vi "Sync Project.vi"() -> ()   [LabVIEW 2011, in "LVH-Build-Tools.lvlib"]
doc: "This VI duplicates the install directories folder hierarchy in the source directory (if neccissary) and creates hard links in the source directory for each new file in the install directory. This VI should be run each time after LabVIEW development, before checking in code."
uses:
  <vilib>/LabVIEW Hacker/Build Tools/LVH-Build-Tools.lvlib
  vi.lib/LabVIEW Hacker/Build Tools/Private/Type Defs/Sync Source State.ctl
panel:
  out "Error Out":errorcluster
  out "Window":enum32{"Init", "Configure", "Sync", "Summary"}(tab)
  in  "Config Help Button":bool
  in  "Settings Button":bool
  in  "Project":u16(ring) items=["LVH-Adept", "LVH-Build-Tools", "LVH-LINX", "LVH-Revert", "LVH-Toolbox"]
  in  "LabVIEW Version":u16(ring) items=["NI LabVIEW 2011 SP1"]
  in  "Config Next Button":bool
  in  "Config Cancel":bool
  out "Progress":picture
  out "Mass Compile Log":string
  out "Added Files":string[](array[string])
  in  "Summary Finish Button":bool
  out "Deleted Files":string[](array[string])
  out "Archive Link":string
  # "Sync Project\nInitializing..."
  # "Sync Project\n\nPlease choose a project to sync and the version of LabVIEW to sync from."
  # "Sync Project\n\nSyncing, please wait..."
  # "Sync Project\n\nSync complete.  Press Finish to exit."
  # "Backup Archive:"
  # "Mass Compile Log"
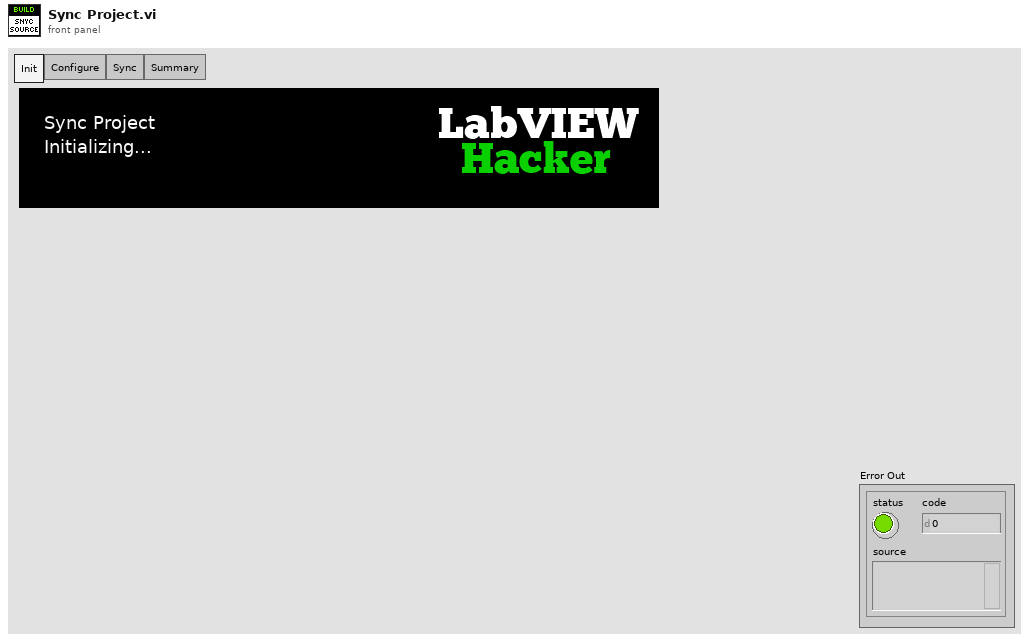
[diagram p1: front panel]
types:
  T1 = typedef "LVH-Build-Tools.lvlib/Sync Source State.ctl" = enum16{"Init", "Configure", "Sync", "Summary"}
  T2 = typedef "LVH-Build-Tools.lvlib/Sync Source Configuration.ctl" = cluster{"Installed Projects":T3[], "Project Source Root Dir":path, "All Config Files":path[], "Selected Project Config":path, "All LabVIEW Dirs":path[], "Selected LabVIEW Dir":path, "Backup Dir":path}
  T3 = typedef "LVH-Build-Tools.lvlib/Installed Project.ctl" = cluster{"Project Name":string, "LV Versions":T4[], "Project Config Path":path}
  T4 = typedef "LVH-Build-Tools.lvlib/_Installed LabVIEW Version.ctl" = cluster{"Version":string, "Path":path}
  T5 = typedef "LVH-Build-Tools.lvlib/_Animation Config.ctl" = cluster{"Image Data":T6[], "Animation Picture Indicator":refnum<vi>, "FPS":u32, "Position":cluster{"X":i16, "Y":i16}}
  T6 = typedef "imagedata.ctl" = cluster{"image type":i32, "image depth":i32, "image":u8[], "mask":u8[], "colors":u32[], "Rectangle":cluster{"left":i16, "top":i16, "right":i16, "bottom":i16}}
  T7 = typedef "LVH-Build-Tools.lvlib/Configuration.ctl" = cluster{"Source Root":path, "Install Root":string, "Components":string[], "Ignore":string[], "Config Files":path[], "LV Directories":path[], "Install Paths":T8}
  T8 = typedef "LVH-Build-Tools.lvlib/Install Configuration.ctl" = cluster{"LabVIEW Directory":path, "Project Source Config":path}
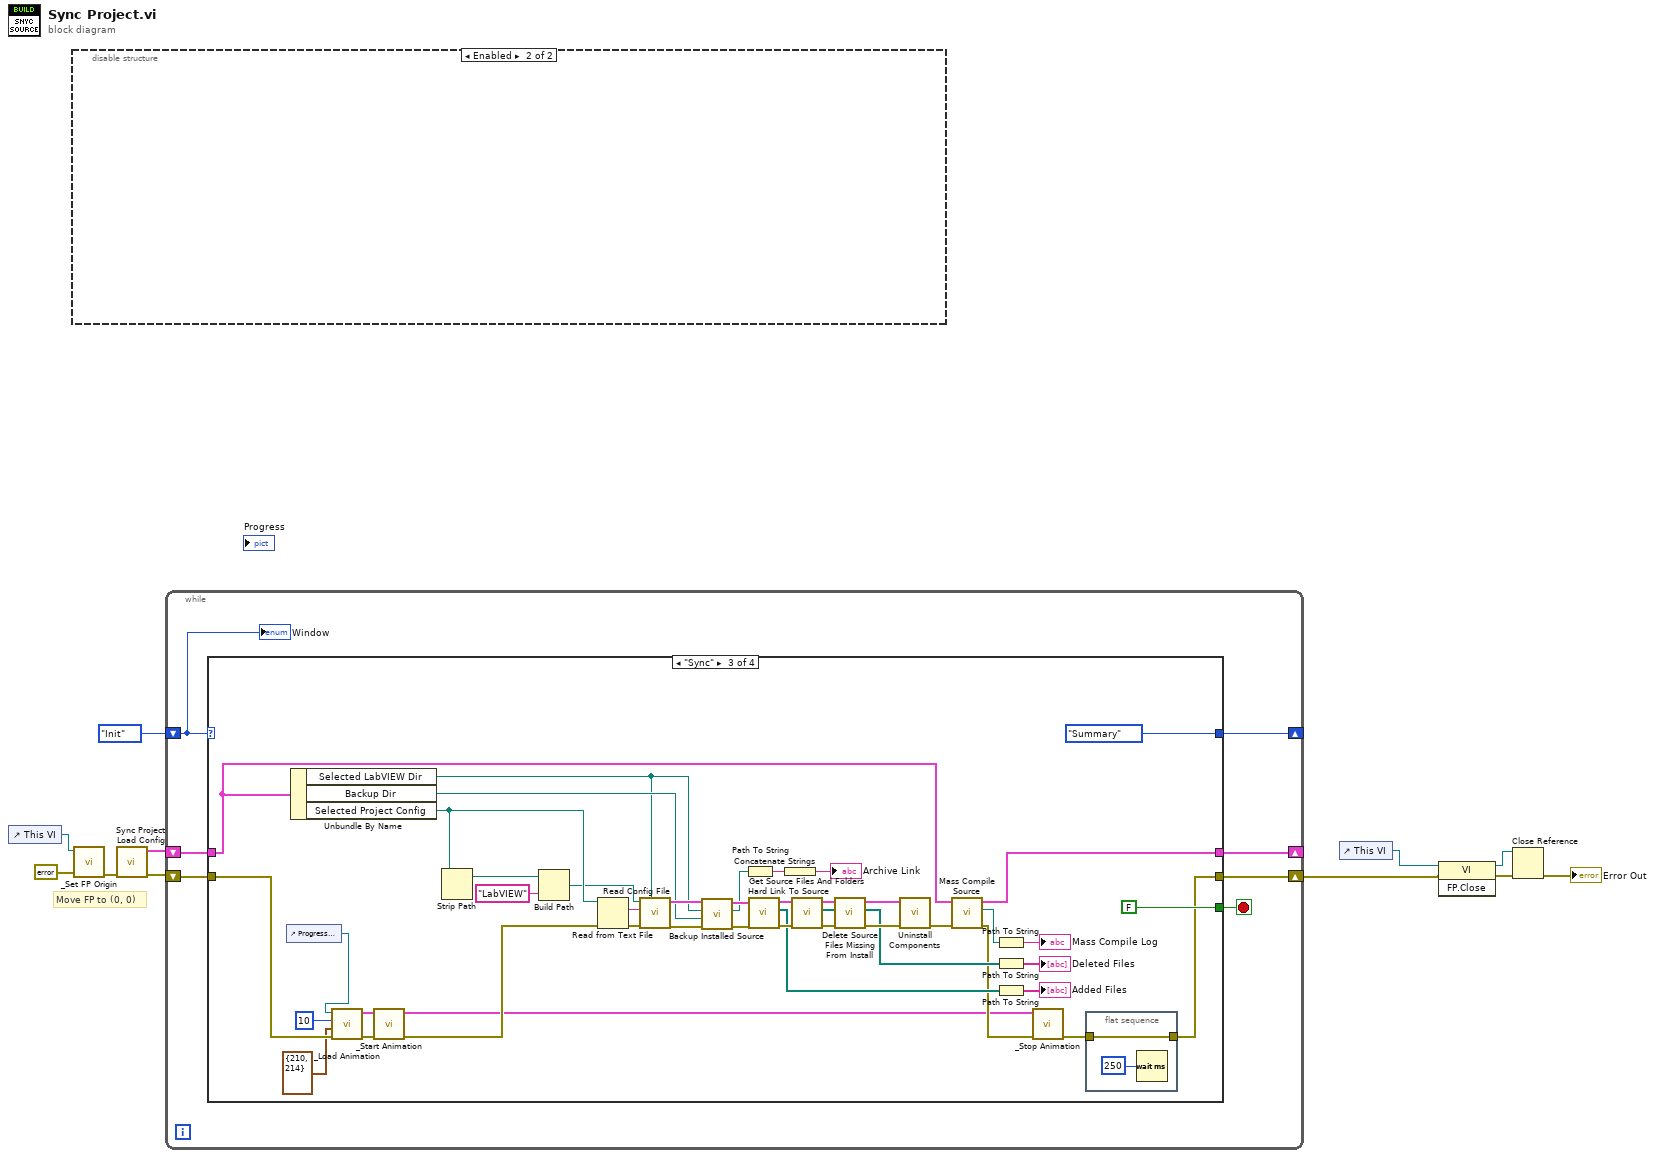
[diagram p0: block diagram]
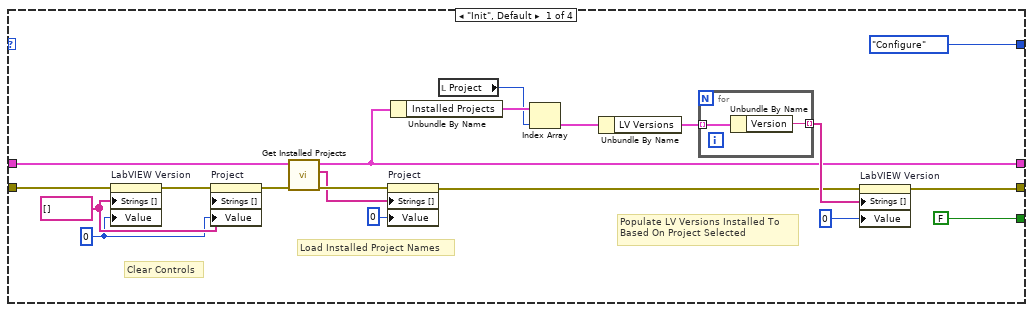
[diagram p2: hidden frame]
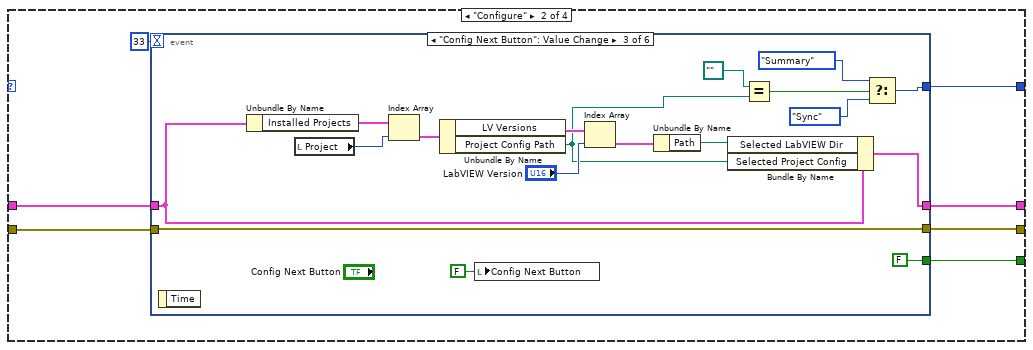
[diagram p3: hidden frame]
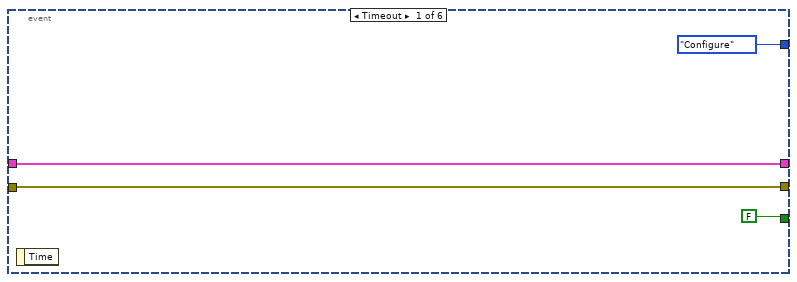
[diagram p4: hidden frame]
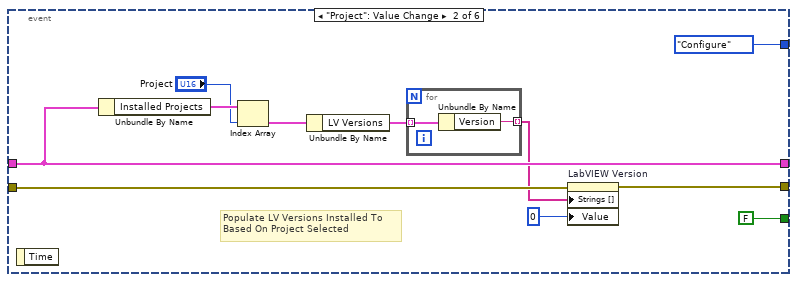
[diagram p5: hidden frame]
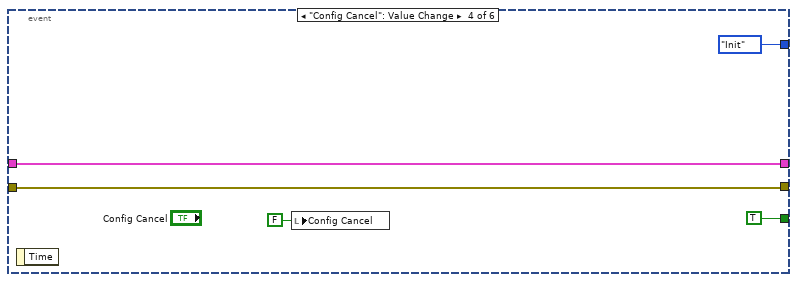
[diagram p6: hidden frame]
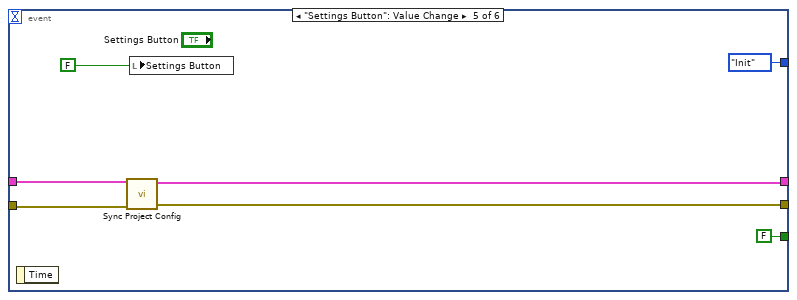
[diagram p7: hidden frame]
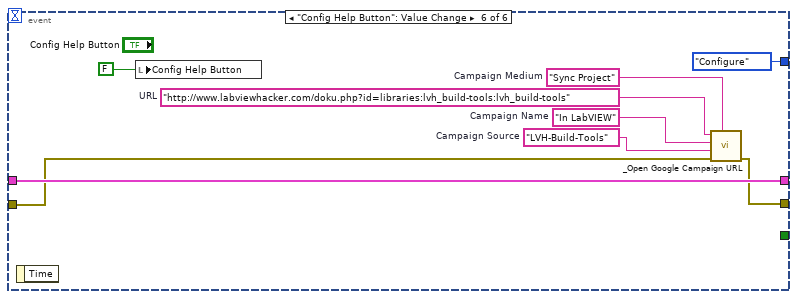
[diagram p8: hidden frame]
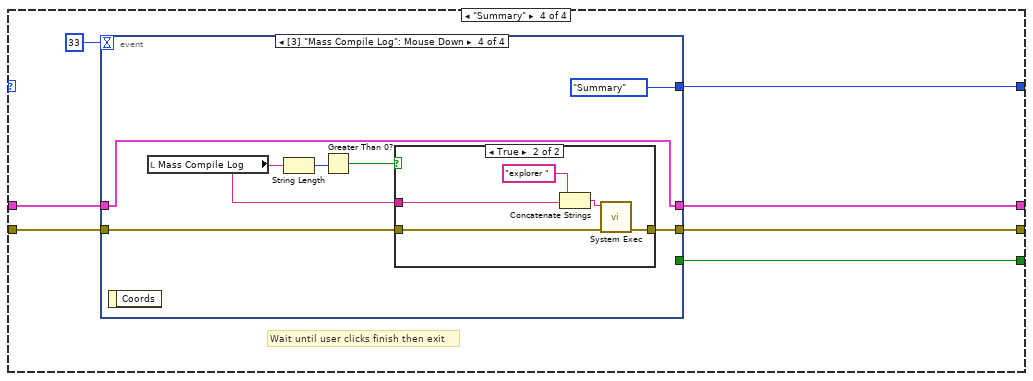
[diagram p9: hidden frame]
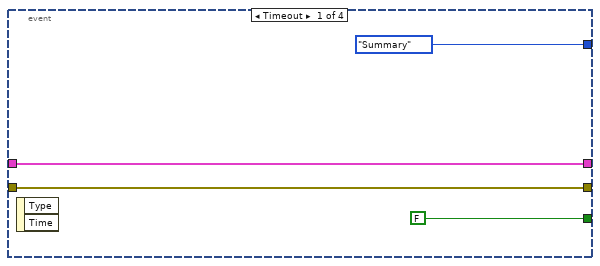
[diagram p10: hidden frame]
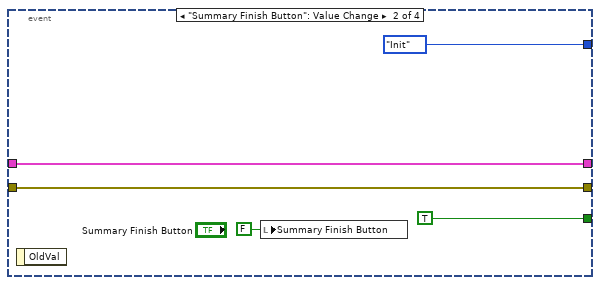
[diagram p11: hidden frame]
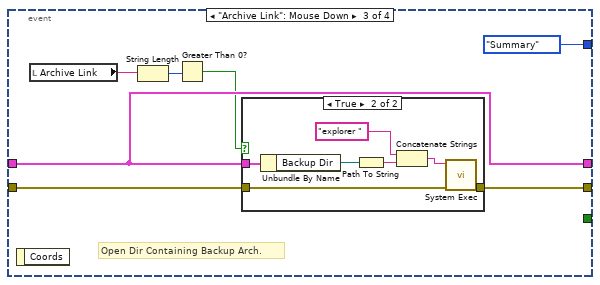
[diagram p12: hidden frame]
diagram:
  # "Move FP to (0, 0)"
  n1 = control-ref of="This VI"() -> (w10:refnum<vi>)
  n2 = disable-structure shown="Enabled" {
    frame Disabled {
    }
    frame Enabled {
    }
  }
  n3 = call "_Set FP Origin.vi"("Error In"=errorcluster {"status"=FALSE, "code"=0, "source"=""} ("Error Out"), "VI Ref"=w10) -> ("Error Out"=w9:errorcluster)  [unwired: 9 in]
  n4 = call "Sync Project Load Config.vi"("Error In"=w9) -> ("Error Out"=w7:errorcluster, "Sync Source Config"=w8:T2)  [unwired: 7 in, 2 out]
  n5 = while {
    shift-right: [w13] -> _
    shift-left: Sync_Source_State."Init" ("Sync Source State") -> [w18]
    shift-right: [w15] -> w1
    shift-left: w7 -> [w17]
    shift-right: [w12] -> _
    shift-left: w8 -> [w16]
    stop <- w14 stop-if-true
    n6 = case shown="\"Sync\"" w18 {
      tunnel: w17 -> [w20 w46 w111 w156]
      tunnel: w16 -> [w19 w44 w122 w151]
      tunnel: [w25 w43 w106 w155] -> w15
      tunnel: [FALSE w45 FALSE w153] -> w14
      tunnel: [Sync_Source_State."Configure" ("Sync Source State") w41 Sync_Source_State."Summary" ("Sync Source State") w150] -> w13
      tunnel: [w27 w42 w121 w152] -> w12
      frame "Init", Default {
        w22 = u16 0
        w23 = string[] [] ("Strings []")
        # "Clear Controls"
        # "Populate LV Versions Installed To \nBased On Project Selected"
        # "Load Installed Project Names"
        n7 = property on="LabVIEW Version" class="Ring (strict)"(error in=w20, "Strings []"=w23, "Value"=w22) -> (error out=w24:errorcluster)  [unwired: 1 in, 1 out]
        n8 = property on="Project" class="Ring (strict)"(error in=w24, "Strings []"=w23, "Value"=w22) -> (error out=w21:errorcluster)  [unwired: 1 in, 1 out]
        n9 = call "Get Installed Projects.vi"("Error In"=w21, "Sync Source Config"=w19) -> ("Error Out"=w36:errorcluster, "Installed Projects"=w35:string[], "Sync Source Config"=w27:T2)  [unwired: 7 in]
        n10 = property on="Project" class="Ring (strict)"(error in=w36, "Strings []"=w35, "Value"=u16 0) -> (error out=w26:errorcluster)  [unwired: 1 in, 1 out]
        n11 = Unbundle By Name(w27) -> ("Installed Projects"=w33:T3[])
        n12 = local read "Project"() -> (w28:u16)
        n13 = Index Array(array=w33, index=w28) -> (element=w32:T3)
        n14 = Unbundle By Name(w32) -> ("LV Versions"=w31:T4[])
        n15 = for {
          tunnel: w31 -> [w40] mode=indexing
          tunnel: [w39] -> w30 mode=indexing
          n16 = Unbundle By Name(w40) -> ("Version"=w39:string)
        }
        n17 = property on="LabVIEW Version" class="Ring (strict)"(error in=w26, "Strings []"=w30, "Value"=u16 0) -> (error out=w25:errorcluster)  [unwired: 1 in, 1 out]
      }
      frame "Configure" {
        n18 = event shown="[2] \"Config Next Button\": Value Change" {
          selector: _ -> [_ _ _ _ _ _]
          dyn-events: _ -> [_ _ _ _ _ _]
          timeout: 33 ("Numeric Control") -> [_ _ _ _ _ _]
          tunnel: w46 -> [w49 w60 w73 w85 w93 w101]
          tunnel: [FALSE FALSE FALSE TRUE FALSE _] -> w45
          tunnel: w44 -> [w50 w56 w78 w84 w92 w103]
          tunnel: [w49 w57 w73 w85 w90 w100] -> w43
          tunnel: [w50 w56 w74 w84 w91 w103] -> w42
          tunnel: [Sync_Source_State."Configure" ("Sync Source State") Sync_Source_State."Configure" ("Sync Source State") w68 Sync_Source_State."Init" ("Sync Source State") Sync_Source_State."Init" ("Sync Source State") Sync_Source_State."Configure" ("Sync Source State")] -> w41
          event Timeout {
            n19 = event-data() -> ()  [unwired: 1 in, 1 out]
          }
          event "Project": Value Change {
            # "Populate LV Versions Installed To \nBased On Project Selected"
            n20 = event-data() -> ()  [unwired: 1 in, 1 out]
            n21 = Unbundle By Name(w56) -> ("Installed Projects"=w62:T3[])
            n22 = Index Array(array=w62, index="Project") -> (element=w59:T3)
            n23 = Unbundle By Name(w59) -> ("LV Versions"=w55:T4[])
            n24 = for {
              tunnel: w55 -> [w64] mode=indexing
              tunnel: [w63] -> w54 mode=indexing
              n25 = Unbundle By Name(w64) -> ("Version"=w63:string)
            }
            n26 = property on="LabVIEW Version" class="Ring (strict)"(error in=w60, "Strings []"=w54, "Value"=u16 0) -> (error out=w57:errorcluster)  [unwired: 1 in, 1 out]
          }
          event "Config Next Button": Value Change {
            n27 = event-data() -> ()  [unwired: 1 in, 1 out]
            n28 = Unbundle By Name(w78) -> ("Installed Projects"=w81:T3[])
            n29 = local read "Project"() -> (w80:u16)
            n30 = Index Array(array=w81, index=w80) -> (element=w79:T3)
            n31 = Unbundle By Name(w79) -> ("LV Versions"=w77:T4[], "Project Config Path"=w65:path)
            n32 = local write "Config Next Button"(FALSE ("Config Next Button")) -> ()
            n33 = Index Array(array=w77, index="LabVIEW Version") -> (element=w75:T4)
            n34 = Unbundle By Name(w75) -> ("Path"=w71:path)
            n35 = Bundle By Name(cluster=w78, "Selected LabVIEW Dir"=w71, "Selected Project Config"=w65) -> (w74:T2)
            n36 = Equal?(x=path "", y=w65) -> (x = y?=w70:bool)
            n37 = Select(t=Sync_Source_State."Summary" ("Sync Source State"), s=w70, f=Sync_Source_State."Sync" ("Sync Source State")) -> (s? t:f=w68:T1)
          }
          event "Config Cancel": Value Change {
            n38 = event-data() -> ()  [unwired: 1 in, 1 out]
            n39 = local write "Config Cancel"(FALSE ("Config Cancel")) -> ()
          }
          event "Settings Button": Value Change {
            n40 = event-data() -> ()  [unwired: 1 in, 1 out]
            n41 = call "Sync Project Config.vi"("Error In"=w93, "Sync Source Config"=w92) -> ("Error Out"=w90:errorcluster, "Sync Source Config"=w91:T2)  [unwired: 8 in]
            n42 = local write "Settings Button"(FALSE ("Settings Button")) -> ()
          }
          event "Config Help Button": Value Change {
            w96 = "LVH-Build-Tools"  # Campaign Source
            w97 = "In LabVIEW"  # Campaign Name
            w98 = "Sync Project"  # Campaign Medium
            w99 = "http://www.labviewhacker.com/doku.php?id=libraries:lvh_build-tools:lvh_build-tools"  # URL
            n43 = event-data() -> ()  [unwired: 1 in, 1 out]
            n44 = local write "Config Help Button"(FALSE ("Help Button")) -> ()
            n45 = call "_Open Google Campaign URL.vi"("Campaign Medium"=w98, "Error In"=w101, "Campaign Source"=w96, "Campaign Name"=w97, "URL"=w99) -> ("Error Out"=w100:errorcluster)  [unwired: 5 in, 1 out]
          }
        }
      }
      frame "Sync" {
        n46 = control-ref of="Progress Animation"() -> (w104:refnum<vi>)
        n47 = Unbundle By Name(w122) -> ("Selected LabVIEW Dir"=w123:path, "Backup Dir"=w124:path, "Selected Project Config"=w116:path)
        n48 = call "_Load Animation.vi"("Error In"=w111, "Position"=cluster{"X":i16, "Y":i16} {"X"=210, "Y"=214}, "FPS"=u32 10, "Animation Picture Indicator"=w104) -> ("Error Out"=w113:errorcluster, "Animation Config"=w114:T5)  [unwired: 6 in]
        n49 = call "_Start Animation.vi"("Error In"=w113, "Animation Config"=w114) -> ("Error Out"=w110:errorcluster, "Animation Config"=w107:T5)  [unwired: 8 in]
        n50 = Strip Path(path=w116) -> (stripped path=w117:path)  [unwired: 1 out]
        n51 = Build Path(base path=w117, name or relative path="LabVIEW") -> (appended path=w115:path)
        n52 = Read from Text File(file (use dialog)=w116, error in=w110) -> (text=w133:string, error out=w132:errorcluster)  [unwired: 2 in, 2 out]
        n53 = call "Read Config File.vi"("LabVIEW Dir Override"=w123, "error in (no error)"=w132, "Config File In"=w133, "Project Source Root"=w115) -> ("error out"=w142:errorcluster, "Configuration out"=w141:T7)  [unwired: 6 in]
        n54 = call "Backup Installed Source.vi"("Error In"=w142, "Backup Dir"=w124, "LabVIEW Dir"=w123, "Configuration"=w141) -> ("Error Out"=w143:errorcluster, "Archive Dest"=w125:path, "Configuration"=w144:T7)  [unwired: 5 in]
        n55 = Path To String(path=w125) -> (string=w127:string)
        n56 = call "Hard Link To Source.vi"("Error In"=w143, "Configuration in"=w144) -> ("Error Out"=w134:errorcluster, "Files Added To Source"=w129:path[], "Configuration out"=w138:T7)  [unwired: 7 in]
        n57 = Concatenate Strings(w127) -> (→"Archive Link":string)
        n58 = call "Get Source Files And Folders.vi"("Error In"=w134, "Configuration"=w138) -> ("Error Out"=w135:errorcluster, "All Source Files"=w137:path[], "Configuration"=w136:T7)  [unwired: 6 in, 1 out]
        n59 = call "Delete Source Files Missing From Install.vi"("Error In"=w135, "Source Files"=w137, "Configuration"=w136) -> ("Error Out"=w139:errorcluster, "Deleted From Souce"=w131:path[], "Configuration"=w140:T7)  [unwired: 6 in]
        n60 = call "Uninstall Components.vi"("Error In"=w139, "Configuration in"=w140) -> ("Error Out"=w145:errorcluster)  [unwired: 7 in, 2 out]
        n61 = call "Mass Compile Source.vi"("Error In"=w145, "Sync Source Config"=w122) -> ("Error Out"=w108:errorcluster, "Mass Compile Log"=w119:path, "Sync Source Config"=w121:T2)  [unwired: 7 in]
        n62 = Path To String(path=w119) -> (string=→"Mass Compile Log":string)
        n63 = Path To String(path=w131) -> (string=→"Deleted Files":string[])
        n64 = Path To String(path=w129) -> (string=→"Added Files":string[])
        n65 = call "_Stop Animation.vi"("Error In"=w108, "Animation Config"=w107) -> ("Error Out"=w105:errorcluster)  [unwired: 9 in]
        n66 = flat-sequence {
          tunnel: [w148] -> w106
          tunnel: w105 -> [w148]
          frame #0 {
            n67 = Wait (ms)(milliseconds to wait=u32 250) -> ()  [unwired: 1 out]
          }
        }
      }
      frame "Summary" {
        # "Wait until user clicks finish then exit"
        n68 = event shown="[3] \"Mass Compile Log\": Mouse Down" {
          selector: _ -> [_ _ _ _]
          dyn-events: _ -> [_ _ _ _]
          timeout: 33 -> [_ _ _ _]
          tunnel: w156 -> [w160 w164 w171 w186]
          tunnel: [w160 w164 w172 w187] -> w155
          tunnel: [FALSE TRUE _ _] -> w153
          tunnel: [w158 w162 w169 w185] -> w152
          tunnel: w151 -> [w158 w162 w169 w185]
          tunnel: [Sync_Source_State."Summary" ("Sync Source State") Sync_Source_State."Init" ("Sync Source State") Sync_Source_State."Summary" ("Sync Source State") Sync_Source_State."Summary" ("Sync Source State")] -> w150
          event Timeout {
            n69 = event-data() -> ()  [unwired: 1 in, 2 out]
          }
          event "Summary Finish Button": Value Change {
            n70 = event-data() -> ()  [unwired: 1 in, 1 out]
            n71 = local write "Summary Finish Button"(FALSE ("Summary Finish Button")) -> ()
          }
          event "Archive Link": Mouse Down {
            # "Open Dir Containing Backup Arch."
            n72 = event-data() -> ()  [unwired: 1 in, 1 out]
            n73 = local read "Archive Link"() -> (w168:string)
            n74 = String Length(string=w168) -> (length=w167:i32)
            n75 = Greater Than 0?(x=w167) -> (x > 0?=w166:bool)
            n76 = case shown="True" w166 {
              tunnel: [w173 w177] -> w172
              tunnel: w171 -> [w173 w176]
              tunnel: w169 -> [_ w174]
              frame False {
              }
              frame True {
                n77 = Unbundle By Name(w174) -> ("Backup Dir"=w175:path)
                n78 = Path To String(path=w175) -> (string=w179:string)
                n79 = Concatenate Strings("explorer " ("string"), w179) -> (w178:string)
                n80 = call <vilib>:"System Exec.vi"("error in (no error)"=w176, "command line"=w178) -> ("error out"=w177:errorcluster)  [unwired: 6 in, 3 out]
              }
            }
          }
          event "Mass Compile Log": Mouse Down {
            n81 = event-data() -> ()  [unwired: 1 in, 1 out]
            n82 = local read "Mass Compile Log"() -> (w181:string)
            n83 = String Length(string=w181) -> (length=w183:i32)
            n84 = Greater Than 0?(x=w183) -> (x > 0?=w182:bool)
            n85 = case shown="True" w182 {
              tunnel: [w188 w191] -> w187
              tunnel: w186 -> [w188 w190]
              tunnel: w181 -> [_ w189]
              frame False {
              }
              frame True {
                n86 = Concatenate Strings("explorer " ("string"), w189) -> (w192:string)
                n87 = call <vilib>:"System Exec.vi"("error in (no error)"=w190, "command line"=w192) -> ("error out"=w191:errorcluster)  [unwired: 6 in, 3 out]
              }
            }
          }
        }
      }
    }
    "Window" <- w18
  }
  n88 = control-ref of="This VI"() -> (w4:refnum<vi>)
  n89 = invoke class="VI" method="FP.Close"(reference=w4, error in=w1) -> (reference out=w3:refnum<vi>, error out=w2:errorcluster)  [unwired: 1 in, 1 out]
  n90 = Close Reference(reference=w3, error in (no error)=w2) -> (error out=→"Error Out":errorcluster)
